vi "WL2Span.vi"(8 "stop":dbl, 11 "start":dbl) -> (0 "span":dbl, 3 "center":dbl)   [LabVIEW 2017]
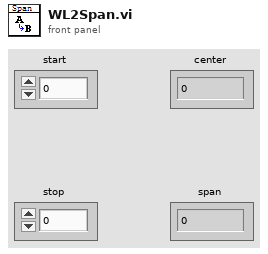
[diagram p1: front panel]
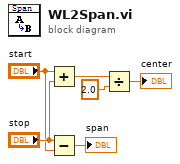
[diagram p0: block diagram]
diagram:
  n1 = Add(x="start", y="stop") -> (x+y=w6:dbl)
  n2 = Subtract(x="stop", y="start") -> (x-y=→"span":dbl)
  n3 = Divide(x=w6, y=2.0) -> (x/y=→"center":dbl)
